vi "caller.vi"() -> ()   [LabVIEW 2024]
uses:
  C:/Users/tupp_js/Documents/LabVIEW Data/Ref Leakds/SMALCLASS/SMALCLASS.lvclass
panel:
  in  "Stop":bool
  out "error out":errorcluster
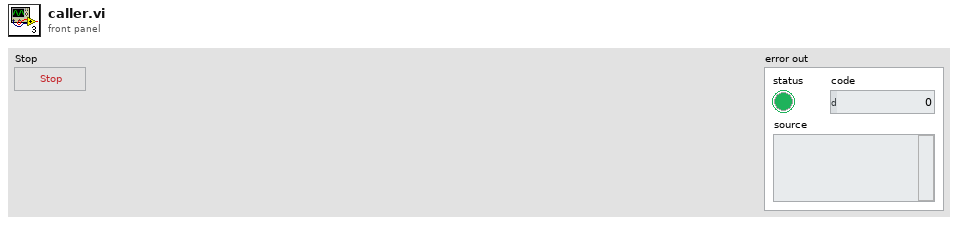
[diagram p1: front panel]
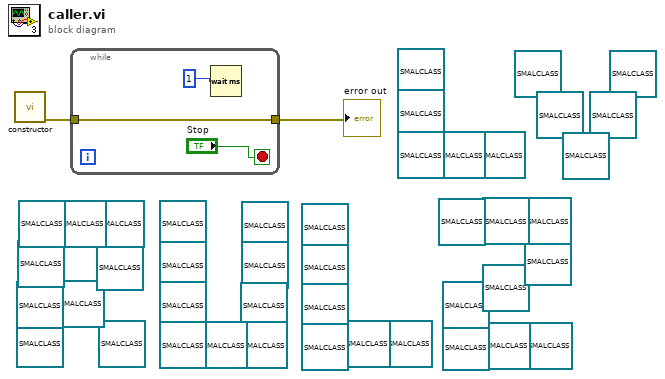
[diagram p0: block diagram]
diagram:
  (unwired) refnum<class "SMALCLASS.lvclass"> refnum ("SMALCLASS.lvclass")
  (unwired) refnum<class "SMALCLASS.lvclass"> refnum ("SMALCLASS.lvclass")
  (unwired) refnum<class "SMALCLASS.lvclass"> refnum ("SMALCLASS.lvclass")
  (unwired) refnum<class "SMALCLASS.lvclass"> refnum ("SMALCLASS.lvclass")
  (unwired) refnum<class "SMALCLASS.lvclass"> refnum ("SMALCLASS.lvclass")
  (unwired) refnum<class "SMALCLASS.lvclass"> refnum ("SMALCLASS.lvclass")
  (unwired) refnum<class "SMALCLASS.lvclass"> refnum ("SMALCLASS.lvclass")
  (unwired) refnum<class "SMALCLASS.lvclass"> refnum ("SMALCLASS.lvclass")
  (unwired) refnum<class "SMALCLASS.lvclass"> refnum ("SMALCLASS.lvclass")
  (unwired) refnum<class "SMALCLASS.lvclass"> refnum ("SMALCLASS.lvclass")
  (unwired) refnum<class "SMALCLASS.lvclass"> refnum ("SMALCLASS.lvclass")
  (unwired) refnum<class "SMALCLASS.lvclass"> refnum ("SMALCLASS.lvclass")
  (unwired) refnum<class "SMALCLASS.lvclass"> refnum ("SMALCLASS.lvclass")
  (unwired) refnum<class "SMALCLASS.lvclass"> refnum ("SMALCLASS.lvclass")
  (unwired) refnum<class "SMALCLASS.lvclass"> refnum ("SMALCLASS.lvclass")
  (unwired) refnum<class "SMALCLASS.lvclass"> refnum ("SMALCLASS.lvclass")
  (unwired) refnum<class "SMALCLASS.lvclass"> refnum ("SMALCLASS.lvclass")
  (unwired) refnum<class "SMALCLASS.lvclass"> refnum ("SMALCLASS.lvclass")
  (unwired) refnum<class "SMALCLASS.lvclass"> refnum ("SMALCLASS.lvclass")
  (unwired) refnum<class "SMALCLASS.lvclass"> refnum ("SMALCLASS.lvclass")
  (unwired) refnum<class "SMALCLASS.lvclass"> refnum ("SMALCLASS.lvclass")
  (unwired) refnum<class "SMALCLASS.lvclass"> refnum ("SMALCLASS.lvclass")
  (unwired) refnum<class "SMALCLASS.lvclass"> refnum ("SMALCLASS.lvclass")
  (unwired) refnum<class "SMALCLASS.lvclass"> refnum ("SMALCLASS.lvclass")
  (unwired) refnum<class "SMALCLASS.lvclass"> refnum ("SMALCLASS.lvclass")
  (unwired) refnum<class "SMALCLASS.lvclass"> refnum ("SMALCLASS.lvclass")
  (unwired) refnum<class "SMALCLASS.lvclass"> refnum ("SMALCLASS.lvclass")
  (unwired) refnum<class "SMALCLASS.lvclass"> refnum ("SMALCLASS.lvclass")
  (unwired) refnum<class "SMALCLASS.lvclass"> refnum ("SMALCLASS.lvclass")
  (unwired) refnum<class "SMALCLASS.lvclass"> refnum ("SMALCLASS.lvclass")
  (unwired) refnum<class "SMALCLASS.lvclass"> refnum ("SMALCLASS.lvclass")
  (unwired) refnum<class "SMALCLASS.lvclass"> refnum ("SMALCLASS.lvclass")
  (unwired) refnum<class "SMALCLASS.lvclass"> refnum ("SMALCLASS.lvclass")
  (unwired) refnum<class "SMALCLASS.lvclass"> refnum ("SMALCLASS.lvclass")
  (unwired) refnum<class "SMALCLASS.lvclass"> refnum ("SMALCLASS.lvclass")
  (unwired) refnum<class "SMALCLASS.lvclass"> refnum ("SMALCLASS.lvclass")
  (unwired) refnum<class "SMALCLASS.lvclass"> refnum ("SMALCLASS.lvclass")
  (unwired) refnum<class "SMALCLASS.lvclass"> refnum ("SMALCLASS.lvclass")
  (unwired) refnum<class "SMALCLASS.lvclass"> refnum ("SMALCLASS.lvclass")
  (unwired) refnum<class "SMALCLASS.lvclass"> refnum ("SMALCLASS.lvclass")
  (unwired) refnum<class "SMALCLASS.lvclass"> refnum ("SMALCLASS.lvclass")
  (unwired) refnum<class "SMALCLASS.lvclass"> refnum ("SMALCLASS.lvclass")
  (unwired) refnum<class "SMALCLASS.lvclass"> refnum ("SMALCLASS.lvclass")
  n1 = call "constructor.vi"() -> ("error out"=w2:errorcluster)  [unwired: 10 in, 1 out]
  n2 = while {
    tunnel: w2 -> [w5]
    tunnel: [w5] -> w1
    stop <- "Stop" stop-if-true
    n3 = Wait (ms)(milliseconds to wait=u32 1) -> ()  [unwired: 1 out]
  }
  "error out" <- w1
